vi "RTS Set Chamber Conditions.vi"(8 "Error In":errorcluster, 10 "Index":i32, 11 "Chamber 1-1":T1 {"Start Time" format="%<%X\n%x>T"; "End Time" format="%<%X\n%x>T"}) -> (0 "Error Out":errorcluster, 3 "Send Chamber Conditions":bool)   [LabVIEW 2016]
uses:
  Type Definitions/RTS Door Ops Client.ctl
  Type Definitions/RTS Door Opening Schedule.ctl
  Type Definitions/RTS Door Ops Sequence.ctl
panel:
  # "Chamber Conditions:"
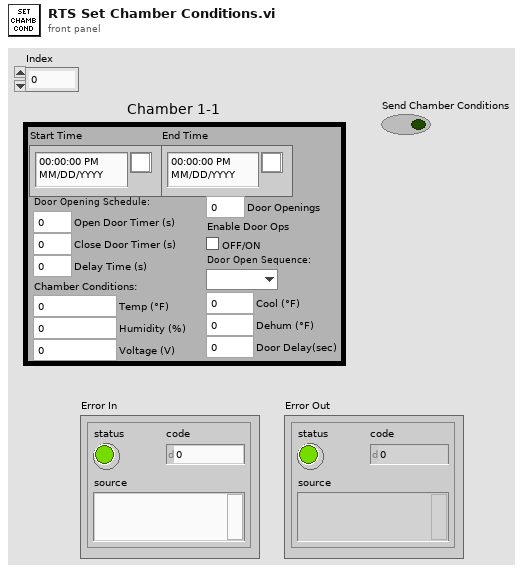
[diagram p1: front panel]
types:
  T1 = typedef "RTS Door Ops Client.ctl" = cluster{"End Time":timestamp, "Start Time":timestamp, "Door Opening Schedule:":T2, "Enable Door Ops":bool, "Door Openings":u32, "Temp (°F)":dbl, "Humidity (%)":dbl, "Voltage (V)":dbl, "Door Open Sequence:":T3, "Door Delay(sec)":dbl, "Dehum (°F)":dbl, "Cool (°F)":dbl}
  T2 = typedef "RTS Door Opening Schedule.ctl" = cluster{"Open Door Timer (s)":dbl, "Delay Time (s)":dbl, "Close Door Timer (s)":dbl}
  T3 = typedef "RTS Door Ops Sequence.ctl" = enum16{"", "1st", "2nd", "3rd"}
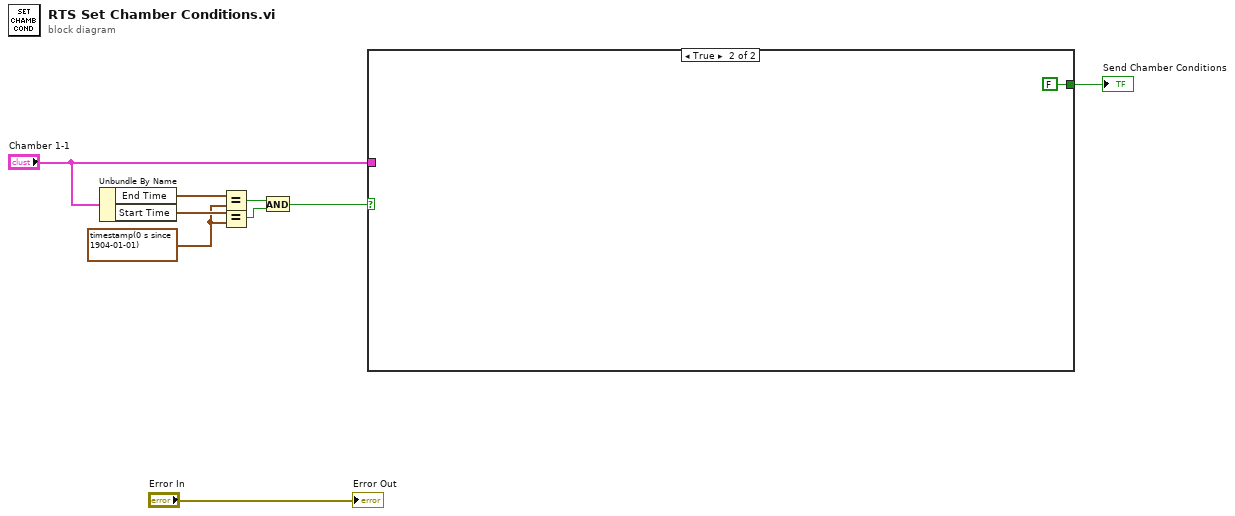
[diagram p0: block diagram]
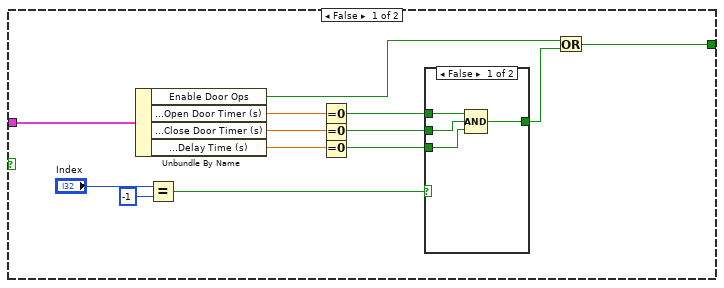
[diagram p2: hidden frame]
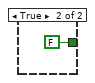
[diagram p3: hidden frame]
diagram:
  w5 = timestamp(0 s since 1904-01-01) ("y")
  n1 = Unbundle By Name("Chamber 1-1") -> ("End Time"=w7:timestamp, "Start Time"=w6:timestamp)
  n2 = Equal?(x=w7, y=w5) -> (x = y?=w4:bool)
  n3 = Equal?(x=w6, y=w5) -> (x = y?=w3:bool)
  n4 = And(x=w4, y=w3) -> (x .and. y?=w2:bool)
  n5 = case shown="True" w2 {
    tunnel: [w22 FALSE] -> w9
    tunnel: "Chamber 1-1" -> [w13 _]
    frame False {
      n6 = Unbundle By Name(w13) -> ("Enable Door Ops"=w21:bool, "Door Opening Schedule:.Open Door Timer (s)"=w14:dbl, "Door Opening Schedule:.Close Door Timer (s)"=w15:dbl, "Door Opening Schedule:.Delay Time (s)"=w16:dbl)
      n7 = Equal?(x="Index", y=-1) -> (x = y?=w10:bool)
      n8 = Equal To 0?(x=w14) -> (x = 0?=w17:bool)
      n9 = Equal To 0?(x=w15) -> (x = 0?=w18:bool)
      n10 = Equal To 0?(x=w16) -> (x = 0?=w19:bool)
      n11 = case shown="False" w10 {
        tunnel: [w26 FALSE] -> w20
        tunnel: w19 -> [w25 _]
        tunnel: w18 -> [w24 _]
        tunnel: w17 -> [w23 _]
        frame False {
          n12 = Compound Arithmetic op=AND(w23, w24, w25) -> (w26:bool)
        }
        frame True {
        }
      }
      n13 = Or(x=w21, y=w20) -> (x .or. y?=w22:bool)
    }
    frame True {
    }
  }
  "Send Chamber Conditions" <- w9
  "Error Out" <- "Error In"
